vi "Sort Matches.vi"(1 "Filter":string, 2 "Matches":string[](array[string]), 3 "Class Matches":string[](array[string])) -> (0 "Filterd Matches":string[](array[string]))   [LabVIEW 2018]
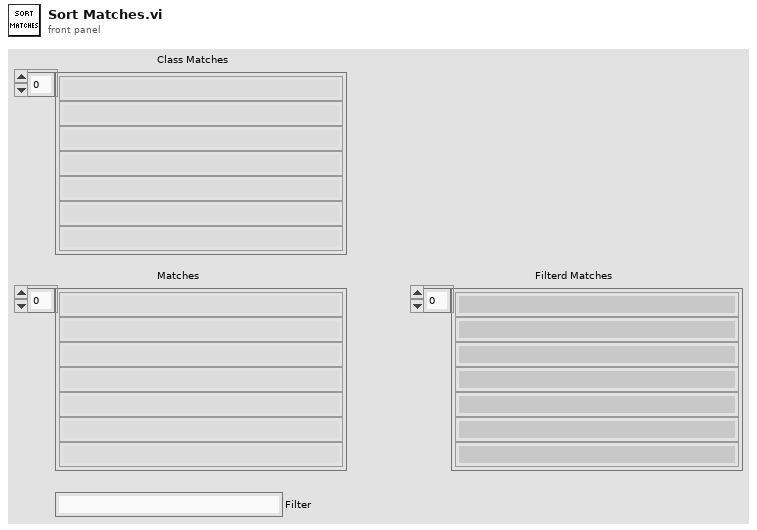
[diagram p1: front panel]
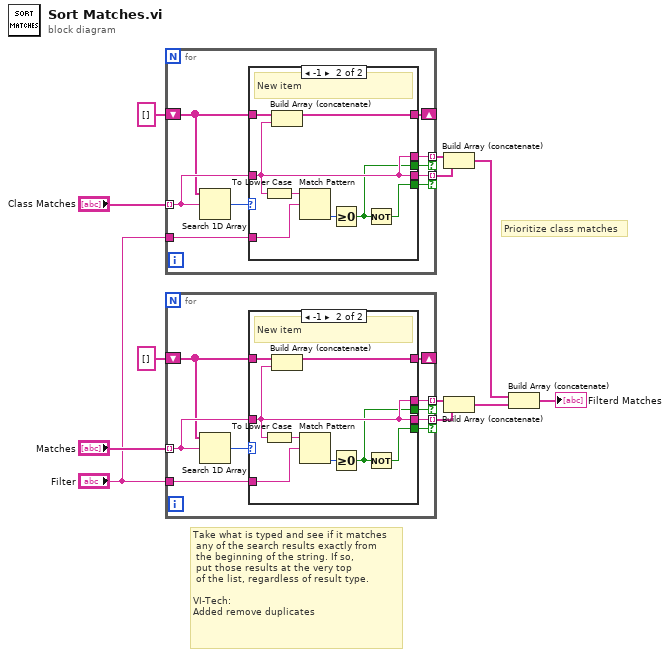
[diagram p0: block diagram]
diagram:
  # "Prioritize class matches"
  # "Take what is typed and see if it matches\n any of the search results exactly from\n the beginning of the string. If so,\n put those results at the very top\n of the list, regardless of result type.\n\nVI-Tech:\nAdded remove duplicates"
  n1 = for {
    tunnel: "Class Matches" -> [w20] mode=indexing
    tunnel: "Filter" -> [w21]
    shift-right: [w18] -> _
    shift-left: string[] [] ("Top match") -> [w17]
    tunnel: [w16] -> w8 mode=indexing if=w13
    tunnel: [w15] -> w7 mode=indexing if=w14
    n2 = Search 1D Array(1D array=w17, element=w20) -> (index of element=w19:i32)  [unwired: 1 in]
    n3 = case shown="-1" w19 {
      tunnel: w20 -> [_ w27]
      tunnel: w21 -> [_ w32]
      tunnel: w17 -> [w24 w30]
      tunnel: [w24 w29] -> w18
      tunnel: [_ w27] -> w16
      tunnel: [_ w27] -> w15
      tunnel: [FALSE w26] -> w14
      tunnel: [FALSE w25] -> w13
      frame Default {
        # "Duplicate item"
      }
      frame -1 {
        # "New item"
        n4 = To Lower Case(string=w27) -> (all lower case string=w31:string)
        n5 = Build Array (concatenate)(w30, w27) -> (w29:string[])
        n6 = Match Pattern(string=w31, regular expression=w32) -> (offset past match=w28:i32)  [unwired: 1 in, 3 out]
        n7 = Greater Or Equal To 0?(x=w28) -> (x >= 0?=w26:bool)
        n8 = Not(x=w26) -> (.not. x?=w25:bool)
      }
    }
  }
  n9 = for {
    tunnel: "Matches" -> [w40] mode=indexing
    tunnel: "Filter" -> [w41]
    shift-right: [w38] -> _
    shift-left: string[] [] ("Top match") -> [w37]
    tunnel: [w36] -> w10 mode=indexing if=w33
    tunnel: [w35] -> w11 mode=indexing if=w34
    n10 = Search 1D Array(1D array=w37, element=w40) -> (index of element=w39:i32)  [unwired: 1 in]
    n11 = case shown="-1" w39 {
      tunnel: w40 -> [_ w47]
      tunnel: w41 -> [_ w52]
      tunnel: w37 -> [w44 w50]
      tunnel: [w44 w49] -> w38
      tunnel: [_ w47] -> w36
      tunnel: [_ w47] -> w35
      tunnel: [FALSE w46] -> w34
      tunnel: [FALSE w45] -> w33
      frame Default {
        # "Duplicate item"
      }
      frame -1 {
        # "New item"
        n12 = To Lower Case(string=w47) -> (all lower case string=w51:string)
        n13 = Build Array (concatenate)(w50, w47) -> (w49:string[])
        n14 = Match Pattern(string=w51, regular expression=w52) -> (offset past match=w48:i32)  [unwired: 1 in, 3 out]
        n15 = Greater Or Equal To 0?(x=w48) -> (x >= 0?=w46:bool)
        n16 = Not(x=w46) -> (.not. x?=w45:bool)
      }
    }
  }
  n17 = Build Array (concatenate)(w7, w8) -> (w2:string[])
  n18 = Build Array (concatenate)(w11, w10) -> (w3:string[])
  n19 = Build Array (concatenate)(w2, w3) -> (→"Filterd Matches":string[])
